vi "Enumerate Ephemeral Strategies.vi"(11 "Platano":refnum<class "Platano.lvclass">) -> (2 "Ephemerals":map{string, refnum<class "BananaPeel.lvclass">}(c390), 3 "Platano":refnum<class "Platano.lvclass">)   [LabVIEW 2021, in "Bananas.lvlib" / "Platano.lvclass"]
uses:
  Platano/Platano.lvclass
  Banana.lvclass
  BananaPeel/BananaPeel.lvclass
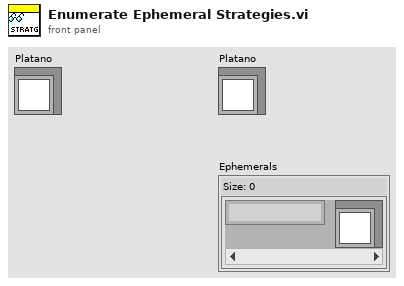
[diagram p1: front panel]
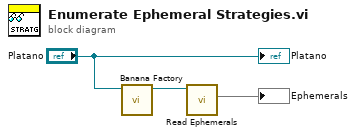
[diagram p0: block diagram]
diagram:
  n1 = call "Banana Factory.vi"("Platano"="Platano") -> ("Banana"=w2:refnum<class "Banana.lvclass">)  [unwired: 10 in]
  n2 = call "Read Ephemerals.vi"("Banana in"=w2) -> ("Ephemerals"=→"Ephemerals":map{string, refnum<class "BananaPeel.lvclass">})  [unwired: 8 in, 2 out]
  "Platano" <- "Platano"
